vi "PB_defines.vi"() -> ()   [LabVIEW 2013]
doc: "This vi is represents the \"defines\" file for the PulseBlaster. It should rarely be changed.\n\nWARNING: Several of the elements consist of information derived from the other elements, but they do not automatically update, (a LabView Global cannot have a functionality), so the user is responsible for keeping things consistent."
panel:
  in  "AI Update Line":u32=4194304 format="%.0x"
  in  "AO Update Line":u32=8388608 format="%.0x"
  in  "Long Delay Time (s)":dbl=42.94967298 format="%.8p"
  in  "Min Instruction Cycle Time (s)":dbl=5e-08 format="%.0p"
  in  "Overhead Time (s)":dbl=3e-08 format="%.0p"
  in  "Clock Period (s)":dbl=1e-08 format="%.0p"
  in  "Long Delay Ticks":u32=4294967295 format="%.0x"
  in  "Min Instruction Ticks":u8=2
  in  "Long Delay Loop Count Correction":u8=2
  in  "Loop Count Correction":u8=1
  in  "Min Delay Loops":u8=3
  in  "Overhead Ticks":u8=3
  in  "Internal Memory Size":u16=512
  in  "External MemorySize":u16=32768
  # "Defined Parameters for Pulse Blaster"
  # "(Period*Long D Ticks)+Overhead time"
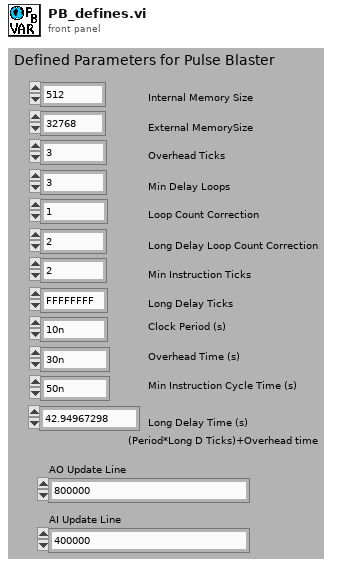
[diagram p1: front panel]
diagram:
